vi "Disconnect.vi"(8 "error in":errorcluster, 11 "DMK33UP2000 in":refnum<class "DMK33UP2000.lvclass">) -> (0 "error out":errorcluster, 3 "DMK33UP2000 out":refnum<class "DMK33UP2000.lvclass">)   [LabVIEW 2018, in "DMK33UP2000.lvlib" / "DMK33UP2000.lvclass"]
uses:
  DMK33UP2000.lvclass
  builds/Camera.lvlibp/Camera.lvclass
  <vilib>/vision/driver/NI_Vision_Acquisition_Software.lvlib
  C:/Users/Ron.Dexter.LUMINARTECH/Desktop/builds/Camera.lvlibp/Camera.lvclass
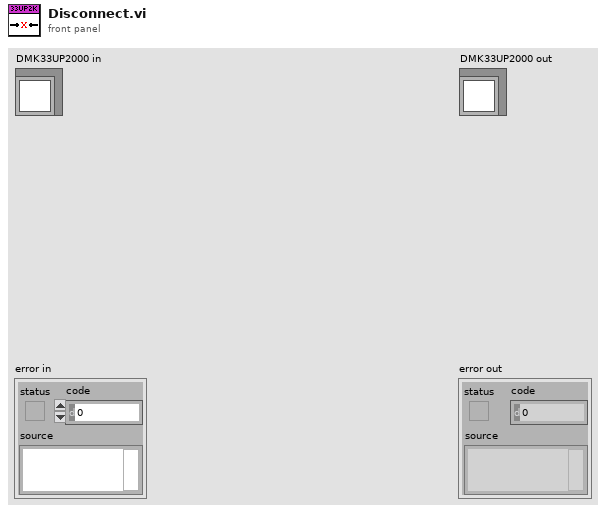
[diagram p1: front panel]
types:
  T1 = typedef "Camera.lvlibp/IMAQdx.ctl" = refnum<k21>
  T2 = typedef "IMAQdx.ctl" = refnum<k21>
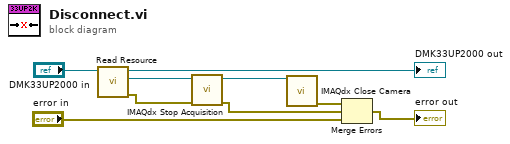
[diagram p0: block diagram]
diagram:
  n1 = call "Read Resource.vi"("Camera in"="DMK33UP2000 in") -> ("error out"=w5:errorcluster, "IMAQdx Session"=w8:T1, "Camera out"=→"DMK33UP2000 out":refnum<class "DMK33UP2000.lvclass">)  [unwired: 8 in]
  n2 = call <vilib>:"IMAQdx Stop Acquisition.vi"("error in"=w5, "Session In"=w8) -> ("error out"=w3:errorcluster, "Session Out"=w7:T2)  [unwired: 8 in]
  n3 = call <vilib>:"IMAQdx Close Camera.vi"("Session In"=w7) -> ("error out"=w4:errorcluster)  [unwired: 10 in]
  n4 = Merge Errors(w4, w3, "error in") -> (→"error out":errorcluster)
